vi "Constants.vi"() -> ()   [LabVIEW 2015, in "Waveform-Processing-Custom-Device Shared.lvlib"]
doc: "Use this Global VI to access the GUIDs assigned to the page resources of the Custom Device."
uses:
  Waveform-Processing-Custom-Device Shared.lvlib
panel:
  in  "Tab Control":enum32{"GUIDS", "Constants", "Properties"}(tab)
  in  "Waveform-Processing-Custom-Device Disabled":string="7b547a45-b3bf-4a70-a525-6bc55fa12b7c"
  in  "Waveform Results Section GUID":string="e38e89f1-3d1b-4012-b75e-d54b3a46b12e"
  in  "Running Average Settings GUID":string="98bae003-a8c4-4cad-9e5d-6f3690f27bc7"
  in  "Waveform-Processing-Custom-Device":string="2e5751d4-f26f-4961-8df7-f46ae00d1276"
  in  "Waveform Processing Custom Device Name":string="Waveform Processing Custom Device"
  in  "Running Average Period":string="Running Average Period"
  in  "Running Average Settings":string="Running Average Settings"
  in  "CD.TaskRate":string="TaskRate"
  in  "CD.BufferSamples":string="BufferSamples"
  in  "CD.TaskDependencyRef":string="TaskDependencyRef"
  in  "CD.BufferSeconds":string="BufferSeconds"
  in  "CD.SelectedWaveforms":string="SelectedWfms"
  in  "CD.AvailableWfms":string="AvailableWfms"
  in  "Result.Section.Single.Point.Channel":string="ResultSinglePoint"
  in  "Running.Average.Settings.Period.Channel":string="RunningAveragePeriod"
  in  "Result.Section.Running.Average.Channel":string="ResultRunningAverage"
  in  "Single.Point.Enabled":string="SinglePointEnabled"
  in  "Running.Average.Enabled":string="RunningAverageEnabled"
  in  "Compiled.Settings":string="CompiledSettings"
  in  "Result.Section.Wfm.Dependency":string="WfmDependency"
  in  "CD.TaskDependency":string="TaskDependency"
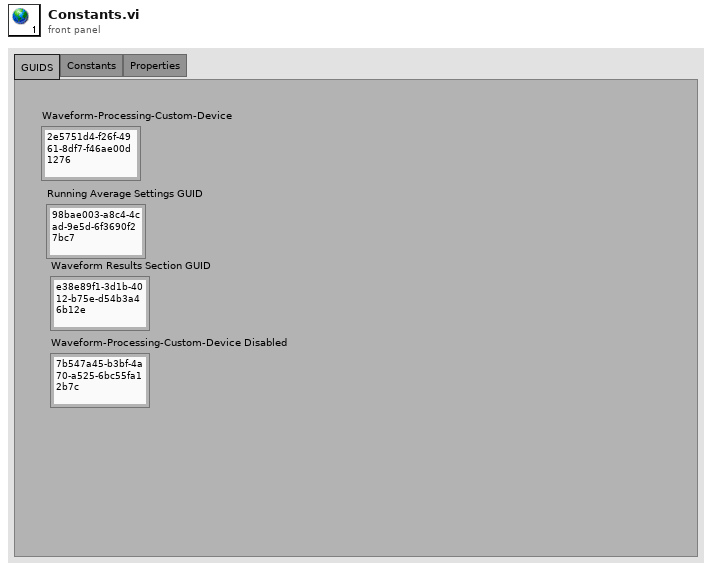
[diagram p1: front panel]
diagram:
